vi "Find Max Constant.vi"(1 "constants":cluster{"a":dbl, "b":dbl, "c":dbl, "d":dbl}) -> (0 "Max or 1":dbl)   [LabVIEW 2016]
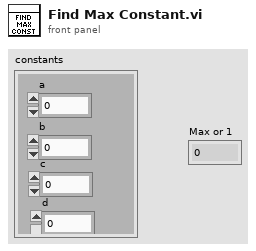
[diagram p1: front panel]
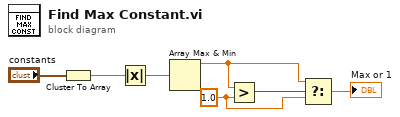
[diagram p0: block diagram]
diagram:
  w5 = 1.0 ("y")
  n1 = Cluster To Array(cluster="constants") -> (array=w2:dbl[])
  n2 = Absolute Value(x=w2) -> (abs(x)=w3:dbl[])
  n3 = Array Max & Min(array=w3) -> (max value=w1:dbl)  [unwired: 3 out]
  n4 = Greater?(x=w1, y=w5) -> (0:w6:bool)
  n5 = Select(t=w1, s=w6, f=w5) -> (s? t:f=→"Max or 1":dbl)
